vi "Create User Defined Steering Frame.vi"(6 "wheel frame angles (rad)":dbl[](array[numeric]), 8 "error in (no error)":errorcluster, 9 "wheel y positions":dbl[](array[numeric]), 10 "wheel x positions":dbl[](array[numeric]), 11 "wheels":refnum<class "NI_Robotics_Wheel.lvclass">[](array[class])) -> (0 "error out":errorcluster, 3 "steering frame out":refnum<class "NI_Robotics_Steering Frame.lvclass">)   [LabVIEW 2017, in "NI_Robotics_Steering Frame.lvclass"]
doc: "Creates a steering frame of the type you specify. You must manually select the polymorphic instance to use."
uses:
  <vilib>/robotics/Steering/Steering Frame/NI_Robotics_Steering Frame.lvclass
  <vilib>/robotics/Steering/Wheel/NI_Robotics_Wheel.lvclass
  <vilib>/robotics/Steering/Wheel/NI_Robotics_Wheel.lvclass/NI_Robotics_Wheel.ctl
  <vilib>/robotics/Steering/Steering Frame/NI_Robotics_Steering Frame.lvclass/NI_Robotics_Steering Frame.ctl
  <vilib>/robotics/Steering/Wheel/Get Wheel Name.vi
  <vilib>/robotics/Steering/Wheel/Update Steering to Wheel Frame Transform.vi
  <vilib>/Analysis/coordinate.llb/Wrap Angle.vi
  <vilib>/Analysis/coordinate.llb/Wrap Angle (array).vi
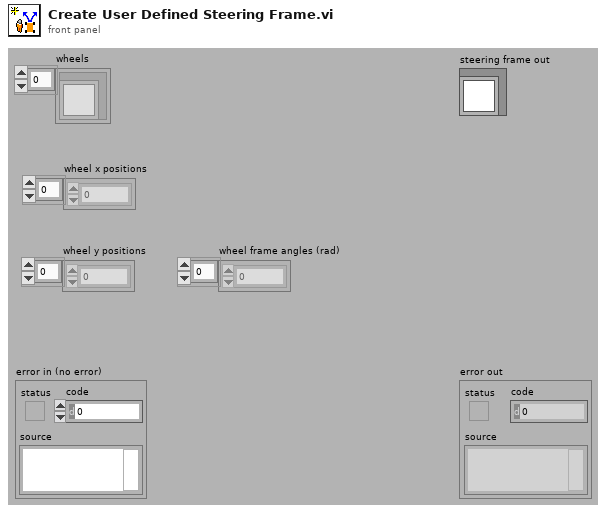
[diagram p1: front panel]
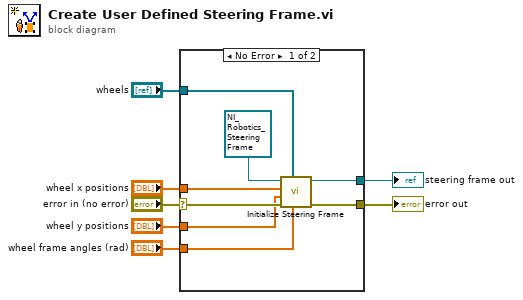
[diagram p0: block diagram]
diagram:
  n1 = case shown="No Error" "error in (no error)" {
    selector: "error in (no error)" -> [w12 w16]
    tunnel: [w10 w16] -> w6
    tunnel: "wheels" -> [w14 _]
    tunnel: "wheel x positions" -> [w13 _]
    tunnel: "wheel frame angles (rad)" -> [w8 _]
    tunnel: "wheel y positions" -> [w9 _]
    tunnel: [w11 _] -> w1
    frame No Error {
      n2 = call <vilib>:"Initialize Steering Frame.vi"("wheel frame angles (rad)"=w8, "wheels"=w14, "error in (no error)"=w12, "wheel y positions"=w9, "wheel x positions"=w13, "steering frame in"=refnum<class "NI_Robotics_Steering Frame.lvclass"> refnum ("Steering Frame in")) -> ("error out"=w10:errorcluster, "steering frame out"=w11:refnum<class "NI_Robotics_Steering Frame.lvclass">)  [unwired: 4 in]
    }
    frame Error {
    }
  }
  "error out" <- w6
  "steering frame out" <- w1
